vi "Teleop.vi"(10 "Match Info":T1={"Autonomous Elapsed Seconds"=0.0, "TeleOp Elapsed Seconds"=0.0, "Disabled Elapsed Seconds"=0.0, "Visited Autonomous"=FALSE, "Visited TeleOp"=FALSE, "Visited Disabled"=FALSE, "Autonomous Settings"={"Autonomous Style"=enum."Independent", "VI Refnum"=refnum}}, 11 "Call Context":T2) -> ()   [LabVIEW 2015]
doc: "This VI is called for each TeleOp packet received from the DS where the robot is not disabled. It is often used to read from the joysticks and update I/O or to update setpoints for timed control loops. It should complete and return within 20 milliseconds or it may miss DS packets."
uses:
  <vilib>/Rock Robotics/WPI/DriverStation/WPI_DriverStationDerivedRobotMode.ctl
  <vilib>/Rock Robotics/WPI/DriverStation/WPI_DriverStationMatch Info.ctl
  <vilib>/Rock Robotics/WPI/CAN/TalonSRX/WPI_CANTalonSRX_BrakeOverride.ctl
  <vilib>/Rock Robotics/WPI/Utilities/WPI_GetSetVariantRefNum.vi
  <vilib>/Rock Robotics/Network Tables/SD Write Number.vi
  <vilib>/Rock Robotics/Network Tables/NT Write Number.vi
  <vilib>/Rock Robotics/Network Tables/SD Write Boolean.vi
  navX Library v2/navX Library v2.lvlib
  <vilib>/Rock Robotics/WPI/Solenoid/Deprecated/WPI_SolenoidSetBool.vi
  <vilib>/Rock Robotics/Network Tables/NT Write Boolean.vi
panel:
  in  "Shooter %":dbl min=0.0 max=0.9 step=0.1
  out "Displacement X":dbl
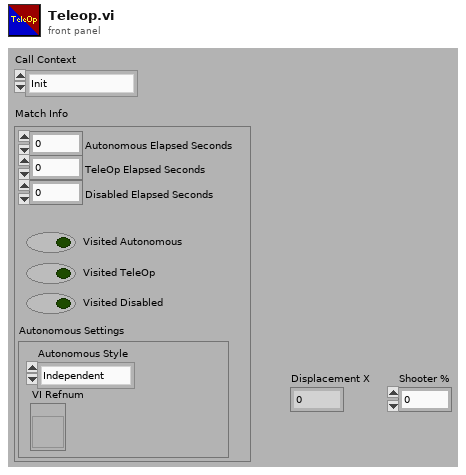
[diagram p1: front panel]
types:
  T1 = typedef "WPI_DriverStationMatch Info.ctl" = cluster{"Autonomous Elapsed Seconds":dbl, "TeleOp Elapsed Seconds":dbl, "Disabled Elapsed Seconds":dbl, "Visited Autonomous":bool, "Visited TeleOp":bool, "Visited Disabled":bool, "Autonomous Settings":cluster{"Autonomous Style":enum16{"Iterative", "Independent"}, "VI Refnum":refnum<vi>}}
  T2 = typedef "WPI_DriverStationDerivedRobotMode.ctl" = enum16{"Init", "Execute", "Stop"}
  T3 = typedef "WPI_CANTalonSRX_BrakeOverride.ctl" = enum8{"No Override", "Override to Coast", "Override to Brake"}
  T4 = typedef "navX Library v2.lvlib/Z900_navX_DeviceTypeDef.ctl" = cluster{"Interface":cluster{"Protocol":T5, "Update Rate (4Hz-60Hz)":u8, "navX Open TypeDef":variant}, "Notify Packet":refnum<notifier>, "Loop VI Refnum":refnum<vi>, "Ready to Close Occurrence Refnum":refnum<k4>}
  T5 = typedef "navX Library v2.lvlib/Z900_navX_ProtocolTypeDef.ctl" = enum16{"SERIAL", "I2C", "SPI"}
  T6 = cluster{"Yaw":dbl, "Roll":dbl, "Pitch":dbl, "Heading":dbl, "Fused Heading":dbl}
  T7 = cluster{"LinearAcceleration X":dbl, "LinearAcceleration Y":dbl, "LinearAcceleration Z":dbl}
  T8 = typedef "WPI_JoystickDevRef.ctl" = cluster{"Device":T9}
  T9 = typedef "WPI_JoystickDeviceEnum.ctl" = enum16{"USB 0", "USB 1", "USB 2", "USB 3", "USB 4", "USB 5"}
  T10 = cluster{"Velocity X":dbl, "Velocity Y":dbl, "Velocity Z":dbl, "Displacement X":dbl, "Displacement Y":dbl, "Displacement Z":dbl}
  T11 = cluster{"Axes[0]":dbl, "Axes[1]":dbl, "Axes[2]":dbl, "Axes[3]":dbl, "Axes[4]":dbl, "Axes[5]":dbl, "Axes[6]":dbl, "Axes[7]":dbl, "Axes[8]":dbl}
  T12 = cluster{"Buttons[0]":bool, "Buttons[1]":bool, "Buttons[2]":bool, "Buttons[3]":bool, "Buttons[4]":bool, "Buttons[5]":bool, "Buttons[6]":bool, "Buttons[7]":bool, "Buttons[8]":bool}
  T13 = typedef "WPI_MotorControlDeviceRef.ctl" = cluster{"DeviceStatus":errorcluster, "Type":T14, "PWM":cluster{"PWM Channel":T15, "DeadBand":T16}, "CAN":cluster{"Device Number":u8, "Control Mode":T17, "Semaphore":T18, "Max Vout":dbl, "TalonSRX Control Mode":T19}, "Invert":bool}
  T14 = typedef "WPI_MotorControlType.ctl" = enum16{"PWM", "CAN", "CANTalonSRX"}
  T15 = typedef "FPGA_DIOPWMChannel.ctl" = enum8{"PWM 0", "PWM 1", "PWM 2", "PWM 3", "PWM 4", "PWM 5", "PWM 6", "PWM 7", "PWM 8", "PWM 9", "PWM MXP 0", "PWM MXP 1", "PWM MXP 2", "PWM MXP 3", "PWM MXP 4", "PWM MXP 5", "PWM MXP 6", "PWM MXP 7", "PWM MXP 8", "PWM MXP 9", "Invalid"}
  T16 = typedef "WPI_PWMDeadband.ctl" = cluster{"Name":string, "maxPositivePwm":i32, "minPositivePwm":i32, "centerPwm":i32, "maxNegativePwm":i32, "minNegativePwm":i32, "angularRange":u16}
  T17 = typedef "WPI_CANJaguar_ControlMode.ctl" = enum8{"Percent VBus", "Current", "Speed", "Position", "Voltage"}
  T18 = typedef "Semaphore RefNum" = refnum<k1>
  T19 = typedef "WPI_CANTalonSRX_APIControlMode.ctl" = enum8{"Percent VBus", "Speed", "Position", "Slave", "Unchanged / Invalid", "Voltage Compensation", "Current", "Motion Profile"}
  T20 = typedef "WPI_CANTalonSRX_GlobalStatus.ctl" = cluster{"Applied Throttle":dbl, "Module Enabled":bool, "CAN Error":errorcluster, "Closed Loop Error":dbl, "Forward Limit Switch Closed":bool, "Reverse Limit Switch Closed":bool, "Sensor Position":dbl, "Sensor Velocity":dbl, "Current":dbl, "Sticky Fault - Over Temp":bool, "Sticky Fault - Under Voltage":bool, "Sticky Fault - Forward Limit":bool, "Sticky Fault - Reverse Limit":bool, "Sticky Fault - Forward Soft Limit":bool, "Sticky Fault - Reverse Soft Limit":bool, "Brake is Enabled":bool, "Encoder Position":dbl, "Encoder Velocity":dbl, "Encoder Index Count":dbl, "Encoder A Pin State":bool, "Encoder B Pin State":bool, "Encoder Index Pin State":bool, "Analog In":dbl, "Analog In Velocity":dbl, "Temperature (C)":dbl, "Battery Voltage":dbl, "Control 5 Is Supported":bool, "Current Profile Slot Select":dbl, "Pos Div 8":bool, "Vel Div 4":bool, "Pulse Width Position":i32, "Pulse Width Velocity":i32, "Pulse Width Rise To Rise (us)":i32, "Pulse Width Rise To Fall (us)":i32, "Mot Prof Active Is Under Run":bool, "Mot Prof Active Has Under Run":bool, "Mot Prof Active Is Last":bool, "Mot Prof Active Velocity Only":bool, "Mot Prof Active Is Valid":bool, "Mot Prof Buffer Is Full":bool, "Mot Prof Active Profile Slot Select":i32, "Mot Prof NextID":i32, "Mot Prof Count":i32, "Mot Prof Active Velocity":dbl, "Mot Prof Active Position":dbl, "Mot Prof Output Enable":i32}
  T21 = typedef "WPI_RobotDriveDevRef.ctl" = cluster{"DevStatus":errorcluster, "Motors[]":T13[], "Square Inputs":bool, "Max Output":dbl}
  T22 = typedef "WPI_SolenoidDevRef.ctl" = cluster{"DevStatus":errorcluster, "Pneumatics Control Module":u8, "Forward Solenoid Channel":T23, "Reverse Solenoid Channel":T23}
  T23 = typedef "WPI_SolenoidChannel.ctl" = enum8{"Solenoid 0", "Solenoid 1", "Solenoid 2", "Solenoid 3", "Solenoid 4", "Solenoid 5", "Solenoid 6", "Solenoid 7", "Invalid"}
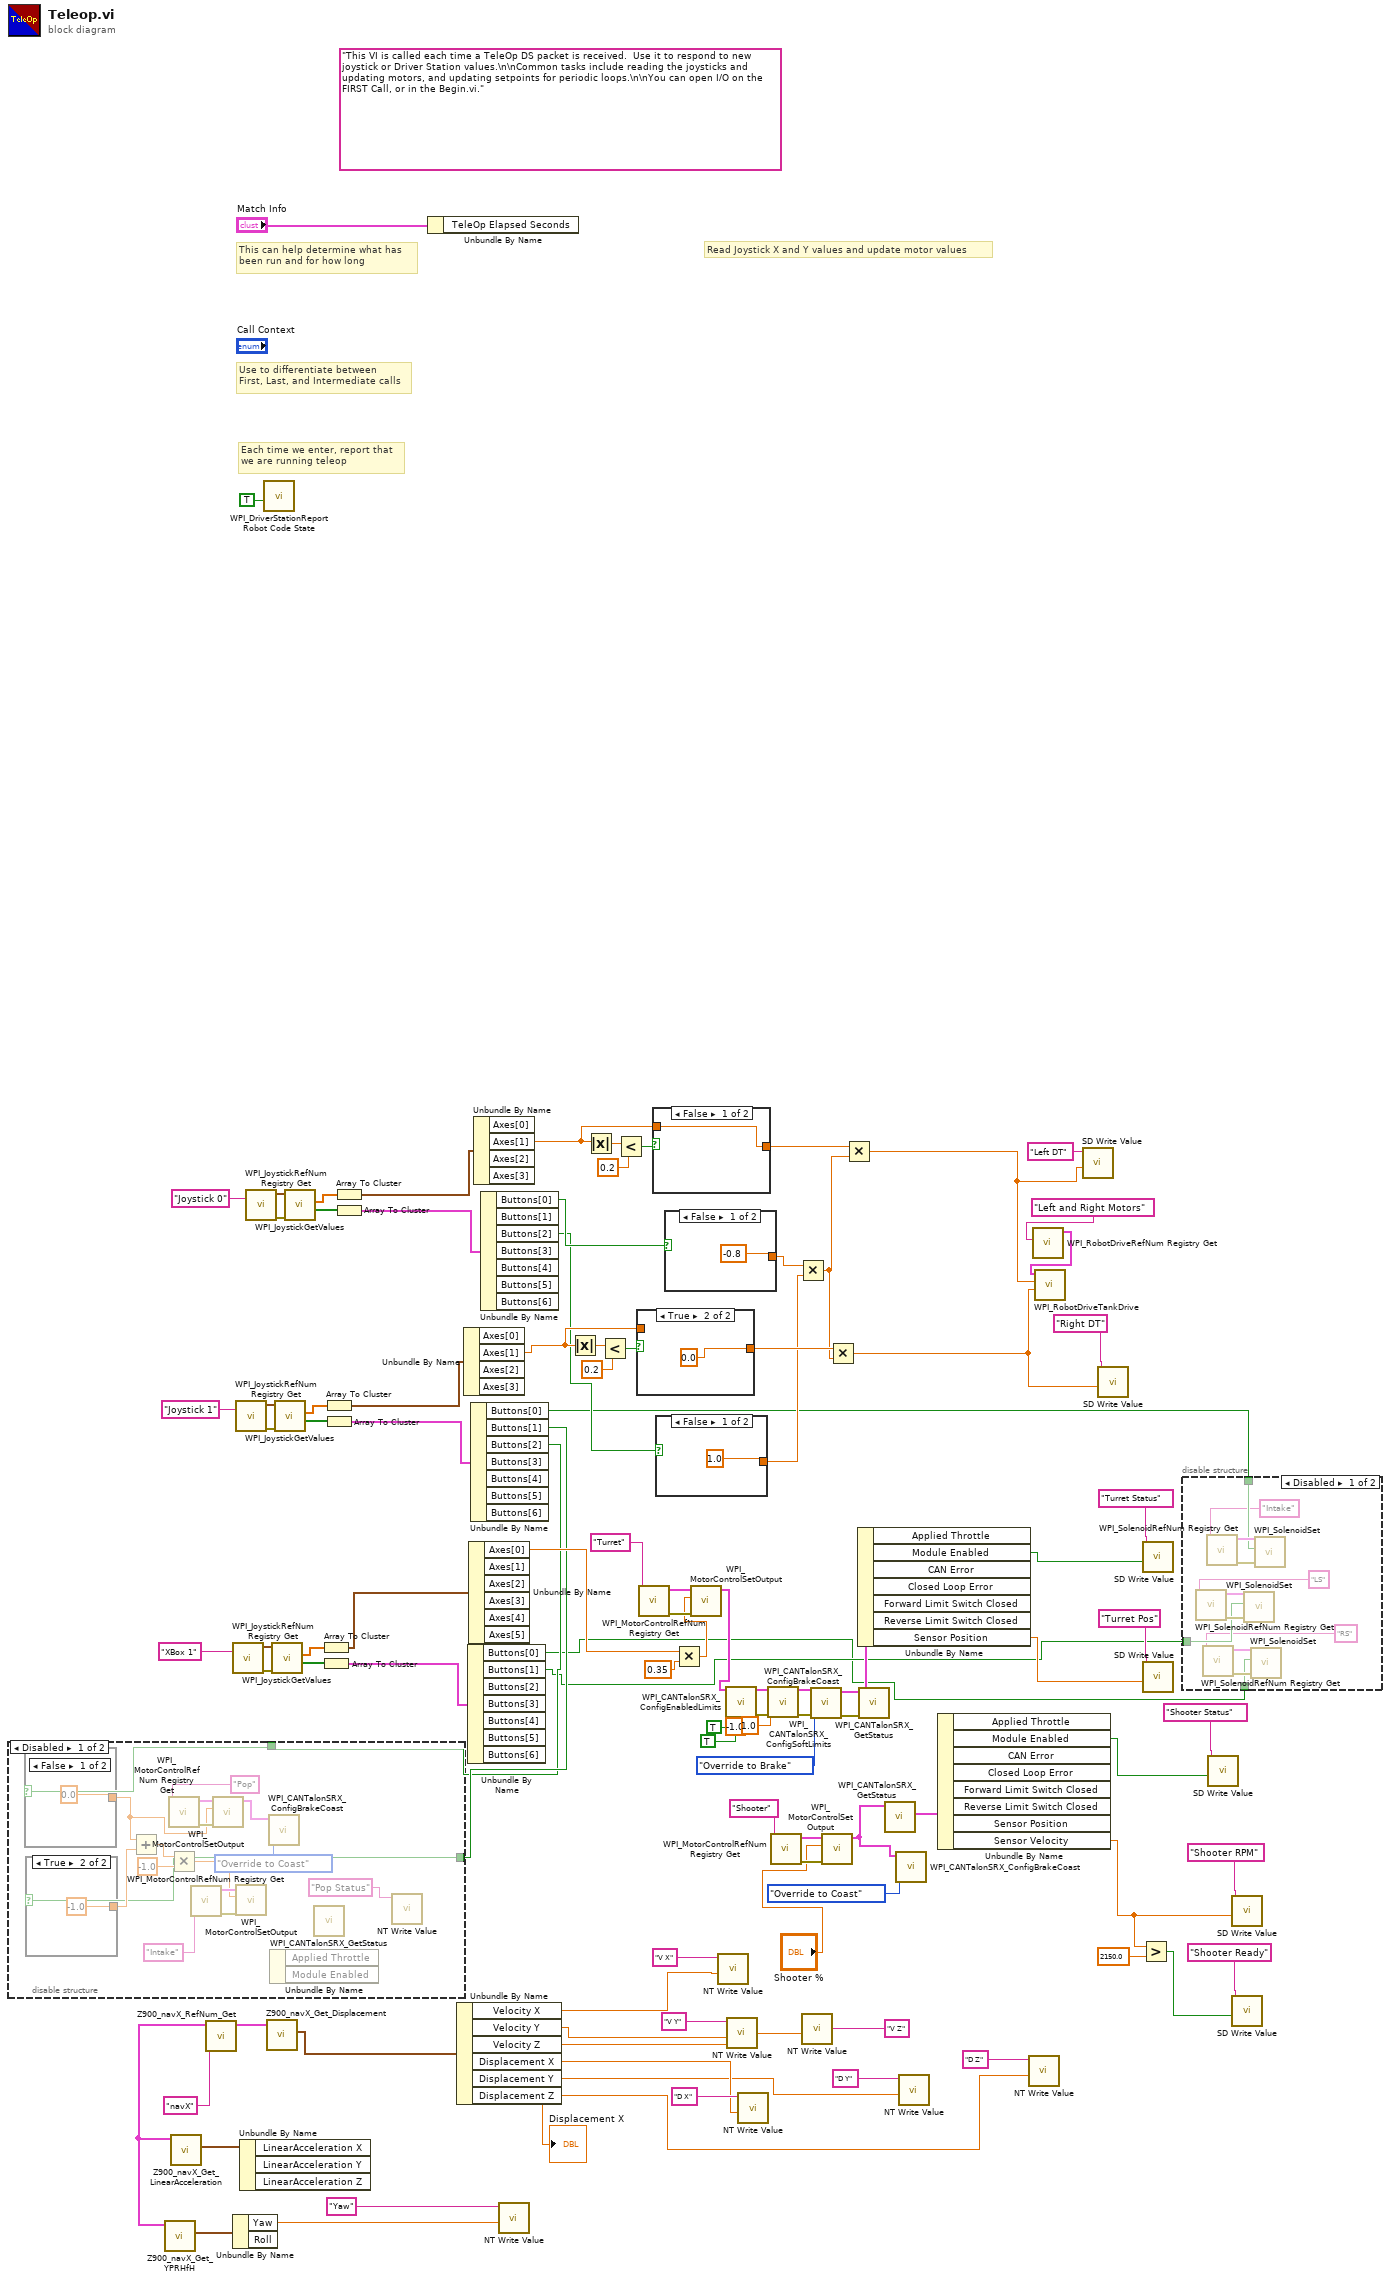
[diagram p0: block diagram]
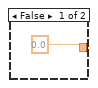
[diagram p3: hidden frame]
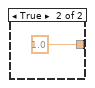
[diagram p4: hidden frame]
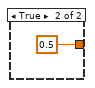
[diagram p6: hidden frame]
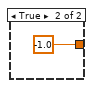
[diagram p7: hidden frame]
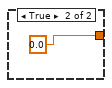
[diagram p9: hidden frame]
diagram:
  (unwired) "This VI is called each time a TeleOp DS packet is received.  Use it to respond to new joystick or Driver Station values.\n\nCommon tasks include reading the joysticks and updating motors, and updating setpoints for periodic loops.\n\nYou can open I/O on the FIRST Call, or in the Begin.vi."
  # "Each time we enter, report that\nwe are running teleop"
  # "Use to differentiate between\nFirst, Last, and Intermediate calls"
  # "This can help determine what has\nbeen run and for how long"
  # "Read Joystick X and Y values and update motor values"
  n1 = call "Z900_navX_RefNum_Get.vi"("refnum name"="navX") -> ("navX Device"=w60:T4)  [unwired: 9 in, 1 out]
  n2 = call "Z900_navX_Get_YPRHfH.vi"("navX Device"=w60) -> ("YRPHfH"=w59:T6)  [unwired: 7 in, 3 out]
  n3 = call "Z900_navX_Get_LinearAcceleration.vi"("navX Device"=w60) -> ("Linear Acceleration"=w67:T7)  [unwired: 7 in, 3 out]
  n4 = call <vilib>:"WPI_JoystickRefNum Registry Get.vi"("refnum name"="XBox 1") -> ("error out"=w49:errorcluster, "JoystickDevRef"=w48:T8)  [unwired: 9 in]
  n5 = Unbundle By Name(w59) -> ("Yaw"=w57:dbl)  [unwired: 1 out]
  n6 = call <vilib>:"WPI_JoystickRefNum Registry Get.vi"("refnum name"="Joystick 1") -> ("error out"=w95:errorcluster, "JoystickDevRef"=w94:T8)  [unwired: 9 in]
  n7 = Unbundle By Name(w67) -> ()  [unwired: 3 out]
  n8 = call <vilib>:"WPI_JoystickRefNum Registry Get.vi"("refnum name"="Joystick 0") -> ("error out"=w102:errorcluster, "JoystickDevRef"=w101:T8)  [unwired: 9 in]
  n9 = call <vilib>:"WPI_DriverStationReport Robot Code State.vi"("TeleOp"=TRUE ("Autonomous")) -> ()  [unwired: 10 in, 1 out]
  n10 = call "Z900_navX_Get_Displacement.vi"("navX Device"=w60) -> ("Displacement"=w75:T10)  [unwired: 7 in, 3 out]
  n11 = call <vilib>:"WPI_JoystickGetValues.vi"("error in (no error)"=w49, "JoystickDevRef"=w48) -> ("Buttons"=w46:bool[], "Axes"=w47:dbl[])  [unwired: 5 in, 3 out]
  n12 = call <vilib>:"WPI_JoystickGetValues.vi"("error in (no error)"=w95, "JoystickDevRef"=w94) -> ("Buttons"=w92:bool[], "Axes"=w93:dbl[])  [unwired: 5 in, 3 out]
  n13 = call <vilib>:"WPI_JoystickGetValues.vi"("error in (no error)"=w102, "JoystickDevRef"=w101) -> ("Buttons"=w99:bool[], "Axes"=w100:dbl[])  [unwired: 5 in, 3 out]
  n14 = Array To Cluster(array=w47) -> (cluster=w45:T11)
  n15 = Array To Cluster(array=w46) -> (cluster=w44:T12)
  n16 = Array To Cluster(array=w93) -> (cluster=w91:T11)
  n17 = Array To Cluster(array=w92) -> (cluster=w90:T12)
  n18 = Array To Cluster(array=w100) -> (cluster=w98:T11)
  n19 = Array To Cluster(array=w99) -> (cluster=w97:T12)
  n20 = Unbundle By Name("Match Info") -> ()  [unwired: 1 out]
  n21 = Unbundle By Name(w75) -> ("Velocity X"=w73:dbl, "Velocity Y"=w71:dbl, "Velocity Z"=w68:dbl, "Displacement X"=w63:dbl, "Displacement Y"=w62:dbl, "Displacement Z"=w61:dbl)
  "Displacement X" <- w63
  n22 = Unbundle By Name(w91) -> ("Axes[1]"=w80:dbl)  [unwired: 3 out]
  n23 = Unbundle By Name(w44) -> ("Buttons[0]"=w4:bool, "Buttons[1]"=w5:bool)  [unwired: 5 out]
  n24 = Unbundle By Name(w45) -> ("Axes[0]"=w39:dbl)  [unwired: 5 out]
  n25 = Unbundle By Name(w90) -> ("Buttons[0]"=w2:bool, "Buttons[1]"=w7:bool, "Buttons[2]"=w6:bool)  [unwired: 4 out]
  n26 = disable-structure shown="Disabled" {
    disable-tunnel: w7 -> [w108 _]
    disable-tunnel: w6 -> [w107 _]
    frame Disabled {
      n27 = case shown="False" w107 {
        tunnel: [0.0 1.0] -> w117
        frame False {
        }
        frame True {
        }
      }
      n28 = case shown="True" w108 {
        tunnel: [0.0 -1.0] -> w124
        frame False {
        }
        frame True {
        }
      }
      n29 = Add(x=w117, y=w124) -> (x+y=w123:dbl)
      n30 = call <vilib>:"WPI_MotorControlRefNum Registry Get.vi"("refnum name"="Pop") -> ("error out"=w121:errorcluster, "MotorControlDevRef"=w120:T13)  [unwired: 9 in]
      n31 = Multiply(x=w123, y=-1.0) -> (x*y=w116:dbl)
      n32 = call <vilib>:"WPI_MotorControlRefNum Registry Get.vi"("refnum name"="Intake") -> ("error out"=w119:errorcluster, "MotorControlDevRef"=w118:T13)  [unwired: 9 in]
      n33 = call <vilib>:"WPI_MotorControlSetOutput.vi"("error in (no error)"=w121, "Output"=w117, "MotorControlDevRef"=w120) -> ("MotorControlDevRef"=w113:T13)  [unwired: 6 in, 2 out]
      n34 = call <vilib>:"WPI_MotorControlSetOutput.vi"("error in (no error)"=w119, "Output"=w116, "MotorControlDevRef"=w118) -> ()  [unwired: 6 in, 3 out]
      n35 = call <vilib>:"WPI_CANTalonSRX_ConfigBrakeCoast.vi"("Brake / Coast Mode"=WPI_CANTalonSRX_BrakeOverride."Override to Coast", "CAN Talon SRX Ref"=w113) -> ("CAN Talon SRX Ref"=w111:T13)  [unwired: 8 in, 1 out]
      n36 = Unbundle By Name() -> (w110:T20, "Module Enabled"=w109)  [unwired: 1 out]
      n37 = call <vilib>:"WPI_CANTalonSRX_GetStatus.vi"() -> ()  [unwired: 9 in, 3 out]
      n38 = call-poly <vilib>:"NT Write Value.vi"("Name"="Pop Status") -> ()  [unwired: 10 in, 1 out]
    }
    frame Enabled {
    }
  }
  n39 = Unbundle By Name(w98) -> ("Axes[1]"=w85:dbl)  [unwired: 3 out]
  n40 = Unbundle By Name(w97) -> ("Buttons[0]"=w54:bool, "Buttons[2]"=w3:bool)  [unwired: 5 out]
  n41 = call-poly <vilib>:"NT Write Value.vi"("Numeric"=w57, "Name"="Yaw") -> ()  [unwired: 9 in, 1 out]
  n42 = Absolute Value(x=w80) -> (abs(x)=w84:dbl)
  n43 = Absolute Value(x=w85) -> (abs(x)=w89:dbl)
  n44 = Less?(x=w84, y=0.2) -> (x < y?=w82:bool)
  n45 = Less?(x=w89, y=0.2) -> (x < y?=w87:bool)
  n46 = case shown="True" w82 {
    tunnel: [w129 0.0] -> w81
    tunnel: w80 -> [w129 _]
    frame False {
    }
    frame True {
    }
  }
  n47 = call <vilib>:"WPI_MotorControlRefNum Registry Get.vi"("refnum name"="Turret") -> ("error out"=w43:errorcluster, "MotorControlDevRef"=w42:T13)  [unwired: 9 in]
  n48 = case shown="False" w87 {
    tunnel: [w131 0.0] -> w86
    tunnel: w85 -> [w131 _]
    frame False {
    }
    frame True {
    }
  }
  n49 = case shown="False" w3 {
    tunnel: [1.0 0.5] -> w52
    frame False {
    }
    frame True {
    }
  }
  n50 = case shown="False" w54 {
    tunnel: [-0.8 -1.0] -> w53
    frame False {
    }
    frame True {
    }
  }
  n51 = Multiply(x=w39, y=0.35) -> (x*y=w38:dbl)
  n52 = call <vilib>:"WPI_MotorControlSetOutput.vi"("error in (no error)"=w43, "Output"=w38, "MotorControlDevRef"=w42) -> ("MotorControlDevRef"=w37:T13)  [unwired: 6 in, 2 out]
  n53 = call-poly <vilib>:"NT Write Value.vi"("Numeric"=w73, "Name"="V X") -> ()  [unwired: 9 in, 1 out]
  n54 = call <vilib>:"WPI_CANTalonSRX_ConfigEnabledLimits.vi"("CAN Talon SRX Ref"=w37, "Forward Soft Limit Enable"=TRUE, "Reverse Soft Limit Enable"=TRUE) -> ("CAN Talon SRX Ref"=w34:T13, "error out"=w33:errorcluster)  [unwired: 11 in]
  n55 = call-poly <vilib>:"NT Write Value.vi"("Numeric"=w71, "Name"="V Y") -> ()  [unwired: 9 in, 1 out]
  n56 = call-poly <vilib>:"NT Write Value.vi"("Numeric"=w63, "Name"="D X") -> ()  [unwired: 9 in, 1 out]
  n57 = call <vilib>:"WPI_CANTalonSRX_ConfigSoftLimits.vi"("CAN Talon SRX Ref"=w34, "Forward Limit Position"=1.0, "Reverse Limit Position"=-1.0, "error in (no error)"=w33) -> ("CAN Talon SRX Ref"=w29:T13, "error out"=w30:errorcluster)  [unwired: 10 in]
  n58 = call <vilib>:"WPI_MotorControlRefNum Registry Get.vi"("refnum name"="Shooter") -> ("error out"=w20:errorcluster, "MotorControlDevRef"=w19:T13)  [unwired: 9 in]
  n59 = Multiply(x=w53, y=w52) -> (x*y=w51:dbl)
  n60 = call-poly <vilib>:"NT Write Value.vi"("Numeric"=w68, "Name"="V Z") -> ()  [unwired: 9 in, 1 out]
  n61 = call <vilib>:"WPI_CANTalonSRX_ConfigBrakeCoast.vi"("error in (no error)"=w30, "Brake / Coast Mode"=WPI_CANTalonSRX_BrakeOverride."Override to Brake", "CAN Talon SRX Ref"=w29) -> ("error out"=w27:errorcluster, "CAN Talon SRX Ref"=w26:T13)  [unwired: 7 in]
  n62 = call <vilib>:"WPI_MotorControlSetOutput.vi"("error in (no error)"=w20, "Output"="Shooter %", "MotorControlDevRef"=w19) -> ("MotorControlDevRef"=w16:T13)  [unwired: 6 in, 2 out]
  n63 = Multiply(x=w81, y=w51) -> (x*y=w55:dbl)
  n64 = Multiply(x=w86, y=w51) -> (x*y=w56:dbl)
  n65 = call <vilib>:"WPI_CANTalonSRX_GetStatus.vi"("error in (no error)"=w27, "CAN Talon SRX Ref"=w26) -> ("Talon SRX Status"=w25:T20)  [unwired: 7 in, 2 out]
  n66 = Unbundle By Name(w25) -> ("Module Enabled"=w23:bool, "Sensor Position"=w21:dbl)  [unwired: 5 out]
  n67 = call <vilib>:"WPI_CANTalonSRX_GetStatus.vi"("CAN Talon SRX Ref"=w16) -> ("Talon SRX Status"=w17:T20)  [unwired: 8 in, 2 out]
  n68 = call <vilib>:"WPI_CANTalonSRX_ConfigBrakeCoast.vi"("Brake / Coast Mode"=WPI_CANTalonSRX_BrakeOverride."Override to Coast", "CAN Talon SRX Ref"=w16) -> ()  [unwired: 8 in, 2 out]
  n69 = call-poly <vilib>:"NT Write Value.vi"("Numeric"=w62, "Name"="D Y") -> ()  [unwired: 9 in, 1 out]
  n70 = Unbundle By Name(w17) -> ("Module Enabled"=w13:bool, "Sensor Velocity"=w10:dbl)  [unwired: 6 out]
  n71 = call-poly <vilib>:"NT Write Value.vi"("Numeric"=w61, "Name"="D Z") -> ()  [unwired: 9 in, 1 out]
  n72 = call <vilib>:"WPI_RobotDriveRefNum Registry Get.vi"("refnum name"="Left and Right Motors") -> ("RobotDriveDevRef"=w79:T21)  [unwired: 9 in, 1 out]
  n73 = call <vilib>:"WPI_RobotDriveTankDrive.vi"("Right axis value"=w55, "Left axis value"=w56, "RobotDriveDevRef"=w79) -> ()  [unwired: 6 in, 3 out]
  n74 = call-poly <vilib>:"SD Write Value.vi"("Numeric"=w56, "Name"="Left DT") -> ()  [unwired: 8 in, 2 out]
  n75 = call-poly <vilib>:"SD Write Value.vi"("Numeric"=w55, "Name"="Right DT") -> ()  [unwired: 8 in, 2 out]
  n76 = Greater?(x=w10, y=2150.0) -> (0:w8:bool)
  n77 = call-poly <vilib>:"SD Write Value.vi"("Boolean"=w23, "Name"="Turret Status") -> ()  [unwired: 8 in, 2 out]
  n78 = call-poly <vilib>:"SD Write Value.vi"("Numeric"=w21, "Name"="Turret Pos") -> ()  [unwired: 8 in, 2 out]
  n79 = disable-structure shown="Disabled" {
    disable-tunnel: w5 -> [w142 _]
    disable-tunnel: w4 -> [w141 _]
    disable-tunnel: w2 -> [w140 _]
    frame Disabled {
      n80 = call <vilib>:"WPI_SolenoidRefNum Registry Get.vi"("refnum name"="LS") -> ("error out"=w146:errorcluster, "SolenoidDevRef"=w145:T22)  [unwired: 9 in]
      n81 = call <vilib>:"WPI_SolenoidRefNum Registry Get.vi"("refnum name"="RS") -> ("error out"=w144:errorcluster, "SolenoidDevRef"=w143:T22)  [unwired: 9 in]
      n82 = call <vilib>:"WPI_SolenoidRefNum Registry Get.vi"("refnum name"="Intake") -> ("error out"=w148:errorcluster, "SolenoidDevRef"=w147:T22)  [unwired: 9 in]
      n83 = call-poly <vilib>:"WPI_SolenoidSet.vi"("error in (no error)"=w146, "Value"=w142, "SolenoidDevRef"=w145) -> ()  [unwired: 7 in, 2 out]
      n84 = call-poly <vilib>:"WPI_SolenoidSet.vi"("error in (no error)"=w144, "Value"=w141, "SolenoidDevRef"=w143) -> ()  [unwired: 7 in, 2 out]
      n85 = call-poly <vilib>:"WPI_SolenoidSet.vi"("error in (no error)"=w148, "Value"=w140, "SolenoidDevRef"=w147) -> ()  [unwired: 7 in, 2 out]
    }
    frame Enabled {
    }
  }
  n86 = call-poly <vilib>:"SD Write Value.vi"("Boolean"=w13, "Name"="Shooter Status") -> ()  [unwired: 8 in, 2 out]
  n87 = call-poly <vilib>:"SD Write Value.vi"("Numeric"=w10, "Name"="Shooter RPM") -> ()  [unwired: 8 in, 2 out]
  n88 = call-poly <vilib>:"SD Write Value.vi"("Boolean"=w8, "Name"="Shooter Ready") -> ()  [unwired: 8 in, 2 out]
